vi "LCV Lookup Valve By Name.vi"(8 "error in (no error)":errorcluster caption="Fehler (Eingang, kein Fehler)", 11 "Valve Name":string) -> (0 "error out":errorcluster caption="Fehler (Ausgang)", 3 "Valve handle":i64)   [LabVIEW 2021, in "labbCAN_Valve_API.lvlib"]
doc: "LCV_Func dev_hdl LCV_CALL LCV_LookupValveByName(const char *pValveName);"
uses:
  labbCAN_Valve_API.lvlib
  labbCAN_Valve_API.dll
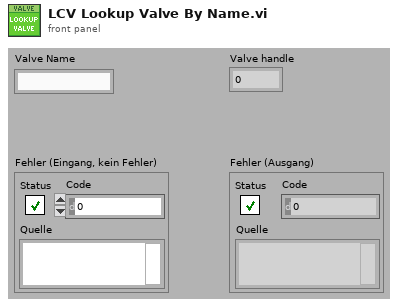
[diagram p1: front panel]
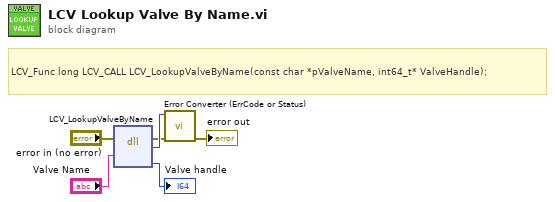
[diagram p0: block diagram]
diagram:
  # "LCV_Func long LCV_CALL LCV_LookupValveByName(const char *pValveName, int64_t* ValveHandle);"
  n1 = dll-call lib="C:/Users/olaja/AppData/Local/CETONI_SDK/labbCAN_Valve_API.*" fn="LCV_LookupValveByName"(error in="error in (no error)", "pValveName"="Valve Name") -> (error out=w3:errorcluster, "Rückgabetyp"=w6:i32, "ValveHandle"=→"Valve handle":i64)  [unwired: 4 in, 1 out]
  n2 = call "Error Converter (ErrCode or Status).vi"("error in (no error)"=w3, "error code"=w6) -> ("error out"=→"error out":errorcluster)  [unwired: 9 in]
